vi "Data_GetType.vi"(8 "error in":errorcluster, 11 "data":variant) -> (0 "error out":errorcluster, 1 "in progress":bool, 2 "type":T1=enum."File", 3 "data out":variant)   [LabVIEW 2017, in "FileManager.lvlib"]
uses:
  <vilib>/addons/InsightCM/Devices/Shared/Common/FileManager/FileManager.lvlib
  <vilib>/addons/InsightCM/Devices/Shared/Common/FileManager/controls/DataType.ctl
  <vilib>/addons/InsightCM/Devices/Shared/Common/FileManager/controls/DataPropertyNames.ctl
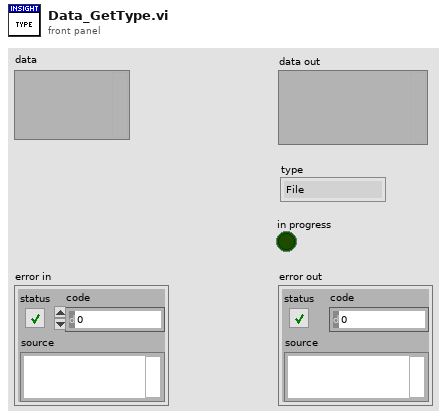
[diagram p1: front panel]
types:
  T1 = typedef "FileManager.lvlib/DataType.ctl" = enum16{"Default", "File", "InMemory", "EventRef", "EventRefFile"}
  T2 = typedef "DataPropertyNames.ctl" = enum16{"Type", "EventRef", "FilePath", "DataGroup", "AcquisitionTimestamp", "StreamId", "StreamBlock", "TrendPointsOnly", "ExtraLargeFile"}
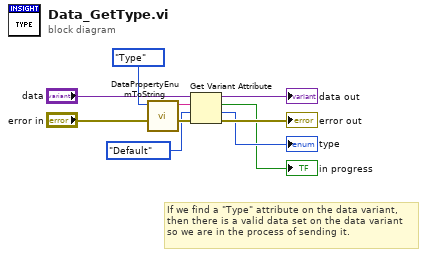
[diagram p0: block diagram]
diagram:
  # "If we find a \"Type\" attribute on the data variant,\nthen there is a valid data set on the data variant\nso we are in the process of sending it."
  n1 = call <vilib>:"DataPropertyEnumToString.vi"("property"=DataPropertyNames."Type" ("Names")) -> ("string"=w7:string)  [unwired: 10 in]
  n2 = Get Variant Attribute(Variant="data", name=w7, default value (empty Variant)=DataType."Default" ("DataType"), error in="error in") -> (duplicate Variant=→"data out":variant, found=→"in progress":bool, value=→"type":T1, error out=→"error out":errorcluster)
